vi "Example Arduino Serial 1.vi"() -> ()   [LabVIEW 2014]
panel:
  in  "Error In":errorcluster
  # "This example will generate code with redefinition structure at beginning,\nneed to manually remove them and after it is OK.\n\ngenerated code code:\n    typedef struct LVcluster_String_String{\n        String LVClusterItem_0;\n        String LVClusterItem_1;\n    };\n\n  /* these two definitions lower needs to be removed */\n\n    typedef struct LVcluster_String_String{    // remove this line\n        String LVClusterItem_0;                         // remove this line\n        String LVClusterItem_1;                         // remove this line\n    };                                                               // remove this line\n    typedef struct LVcluster_String_String{    // remove this line\n        String LVClusterItem_0;                         // remove this line\n        String LVClusterItem_1;                         // remove this line\n    };                                                               // remove this line\n\n    vector<long> shiftRegister_898;\n    bool shiftRegisterInitBool_898 = true;\n\n\n    void Example_Arduino_Serial_1(){\n    long wireUID_696_ = 9600;\n    long wireUID_892_ = 0;\n    vector<LVcluster_String_String> wireUID_845_;\n    LVcluster_String_String wireUID_809_ = {\"three\",\"plum\"};\n    LVcluster_String_String wireUID_803_ = {\"two\",\"orange\"};\n    LVcluster_String_String wireUID_792_ = {\"one\",\"apple\"};\n    wireUID_845_.push_back(wireUID_792_);\n    wireUID_845_.push_back(wireUID_803_);\n    wireUID_845_.push_back(wireUID_809_);\n    Serial.begin(wireUID_696_);\n    /***** BEGIN WhileLoop ********/\n    bool wireUID_2067_ = false; //LoopEndRef.\n    int iteratorUID_180 = 0; //loop iterator\n    do{\n        if (shiftRegisterInitBool_898){\n                            .\n                            .\n                            .\n                 [another code]\n                            .\n                            .\n                            ."
  # "Result should be like after upload to arduino\nusing IDE:"
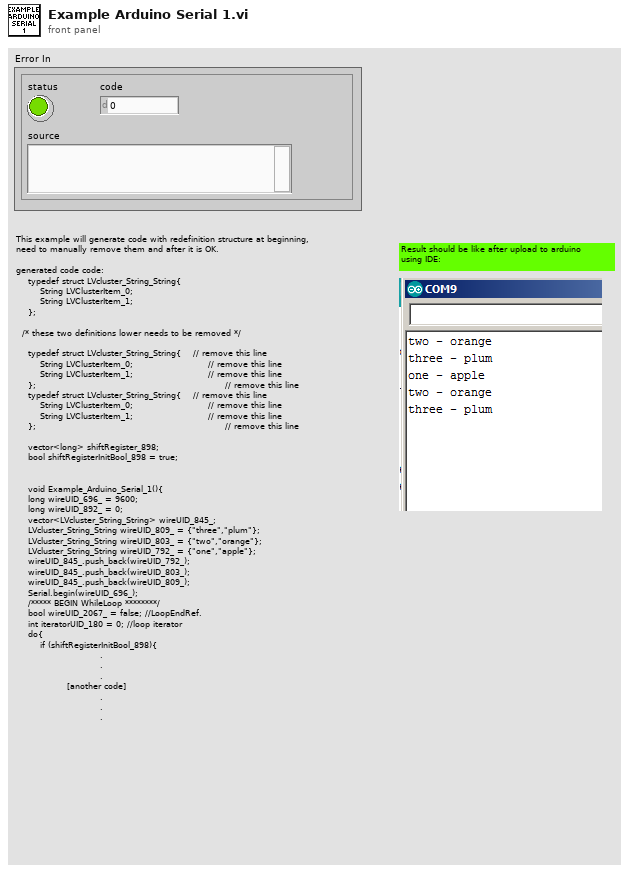
[diagram p1: front panel]
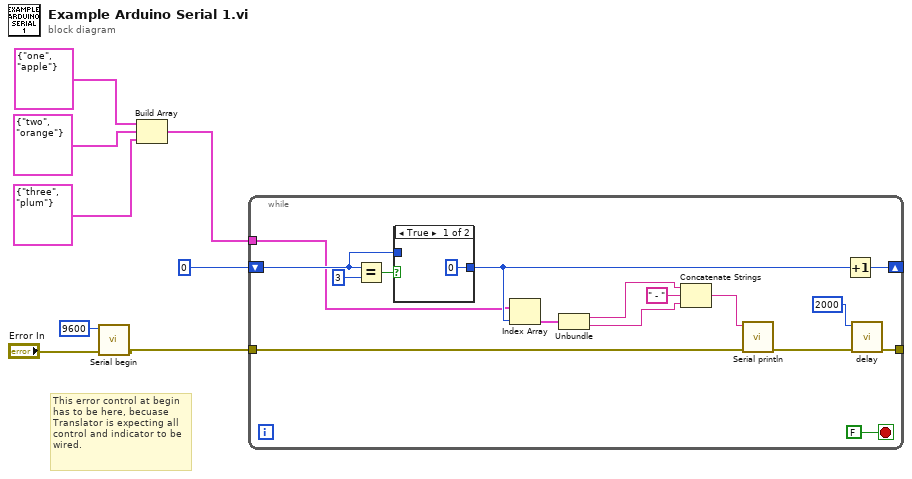
[diagram p0: block diagram]
diagram:
  # "This error control at begin\nhas to be here, becuase Translator is expecting all control and indicator to be wired."
  n1 = call "Serial begin.vi"("Error In"="Error In", "speed (Bd)"=9600) -> ("Error Out"=w3:errorcluster)  [unwired: 9 in]
  n2 = Build Array(cluster{string, string} {"one", "apple"}, cluster{string, string} {"two", "orange"}, cluster{string, string} {"three", "plum"}) -> (w5:cluster{string, string}[])
  n3 = while {
    tunnel: w3 -> [w9]
    tunnel: w5 -> [w19]
    shift-right: [w24] -> _
    shift-left: 0 ("arduino RX pin") -> [w21]
    tunnel: [w16] -> _
    stop <- FALSE stop-if-true
    n4 = Equal?(x=w21, y=3) -> (x = y?=w23:bool)
    n5 = case shown="True" w23 {
      tunnel: w21 -> [_ w26]
      tunnel: [0 ("arduino RX pin") w26] -> w20
      frame True {
      }
      frame False {
      }
    }
    n6 = Index Array(array=w19, index=w20) -> (element=w18:cluster{string, string})
    n7 = Unbundle(w18) -> (w13:string, w12:string)
    n8 = Concatenate Strings(w13, " - " ("String to print"), w12) -> (w11:string)
    n9 = call "Serial println.vi"("Error In"=w9, "string in"=w11) -> ("Error Out"=w10:errorcluster)  [unwired: 9 in]
    n10 = Increment(x=w20) -> (x+1=w24:i32)
    n11 = call "delay.vi"("Error In"=w10, "time (ms)"=2000) -> ("Error Out"=w16:errorcluster)  [unwired: 9 in]
  }
